vi "WLAN Fetch OFDM ModAcc.vi"(0 "Instrument Handle In":refnum<k21>, 1 "Selector String":string, 11 "error in (no error)":errorcluster) -> (4 "Instrument Handle Out":refnum<k21>, 6 "OFDM ModAcc Results":T1 {"Composite Pilot RMS EVM Mean (dB)" format="%.2f"; "Composite Data RMS EVM Mean (dB)" format="%.2f"; "Composite RMS EVM Mean (dB)" format="%.2f"}, 15 "error out":errorcluster)   [LabVIEW 2016, in "RFmxWLAN.lvlib"]
doc: "Fetches common results from the OFDM ModAcc measurement."
uses:
  RFmxWLAN.lvlib
  Typedefs/WLAN OFDM ModAcc Results.ctl
  <vilib>/RFmx/WLAN/mx/RFmxWLAN.llb/RFmxWLAN OFDMModAcc Fetch Composite RMS EVM.vi
  <vilib>/RFmx/WLAN/mx/RFmxWLAN.llb/RFmxWLAN OFDMModAcc Fetch Number of Symbols Used.vi
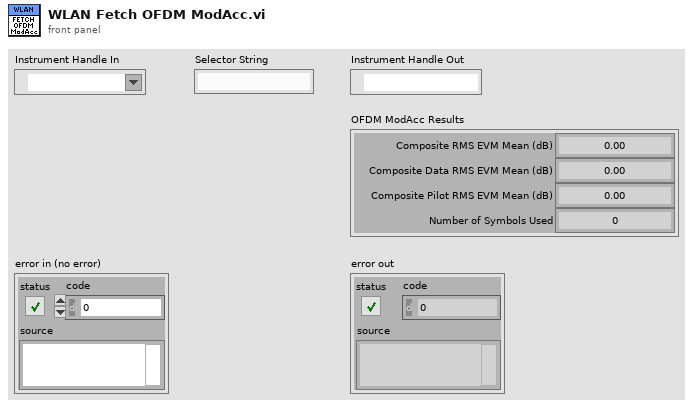
[diagram p1: front panel]
types:
  T1 = typedef "RFmxWLAN.lvlib/WLAN OFDM ModAcc Results.ctl" = cluster{"Composite RMS EVM Mean (dB)":dbl, "Composite Data RMS EVM Mean (dB)":dbl, "Composite Pilot RMS EVM Mean (dB)":dbl, "Number of Symbols Used":i32}
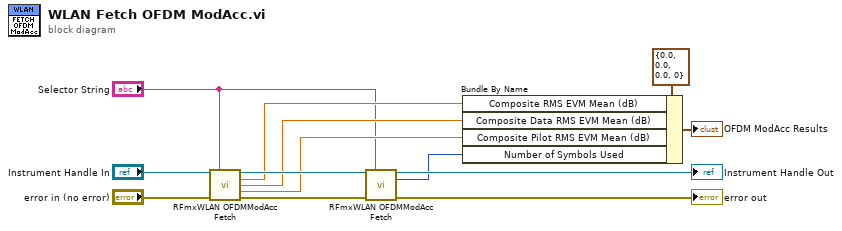
[diagram p0: block diagram]
diagram:
  n1 = call-poly <vilib>:"RFmxWLAN OFDMModAcc Fetch.vi"("Instrument Handle In"="Instrument Handle In", "Selector String"="Selector String", "error in (no error)"="error in (no error)") -> ("Instrument Handle Out"=w8:refnum<k21>, "Composite RMS EVM Mean (dB or %)"=w5:dbl, "Composite Data RMS EVM Mean (dB or %)"=w4:dbl, "Composite Pilot RMS EVM Mean (dB or %)"=w3:dbl, "error out"=w13:errorcluster)  [unwired: 8 in]
  n2 = call-poly <vilib>:"RFmxWLAN OFDMModAcc Fetch.vi"("Instrument Handle In"=w8, "Selector String"="Selector String", "error in (no error)"=w13) -> ("Instrument Handle Out"=→"Instrument Handle Out":refnum<k21>, "Number of Symbols Used"=w2:i32, "error out"=→"error out":errorcluster)  [unwired: 10 in]
  n3 = Bundle By Name(cluster=T1 {"Composite RMS EVM Mean (dB)"=0.0, "Composite Data RMS EVM Mean (dB)"=0.0, "Composite Pilot RMS EVM Mean (dB)"=0.0, "Number of Symbols Used"=0} ("WLAN ModAcc Results"), "Composite RMS EVM Mean (dB)"=w5, "Composite Data RMS EVM Mean (dB)"=w4, "Composite Pilot RMS EVM Mean (dB)"=w3, "Number of Symbols Used"=w2) -> (→"OFDM ModAcc Results":T1)
